vi "POSITION ARM ANGLE.vi"(0 "ARM devref in":T1={"DeviceStatus"={"status"=FALSE, "code"=0, "source"=""}, "Type"=enum."PWM", "PWM"={"PWM Channel"=enum."Invalid", "DeadBand"={"Name"="", "maxPositivePwm"=0, "minPositivePwm"=0, "centerPwm"=0, "maxNegativePwm"=0, "minNegativePwm"=0, "angularRange"=0}}, "CAN"={"Device Number"=0, "SetOutput VI Ref"=variant, "GetOutput VI Ref"=variant, "Enable VI Ref"=variant, "Disable VI Ref"=variant, "Data"=variant}, "Invert"=FALSE, "DIO PWM"={"PWM \"Enable\" Channel"=enum."Invalid", "DIOChannel"=enum."Invalid", "PWM Rate"=0.0}}, 1 "LEFT-RIGHT":string="LEFT", 2 "Setpoint":dbl=515.0, 5 "error in (no error)":errorcluster, 7 "PID Constants":T6={"P Gain"=2.0599999999999987, "I Gain"=0.0, "D Gain"=0.20000000000000004, "F Gain"=0.0, "I Zone"=0.0, "Min Output"=-0.1999999999999993, "Max Output"=0.95} {"Max Output" min=-1.0 max=1.0 step=0.01; "Min Output" min=-1.0 max=1.0 step=0.01; "I Zone" step=0.01; "F Gain" step=0.01; "D Gain" step=0.01; "I Gain" step=0.01; "P Gain" min=0.0 step=0.01}) -> (14 "Position":dbl, 16 "Output":dbl, 19 "error out":errorcluster)   [LabVIEW 2020]
uses:
  <vilib>/Rock Robotics/WPI/MotorControl/WPI_MotorControlDeviceRef.ctl
  <vilib>/Rock Robotics/WPI/MotorControl/WPI_MotorControlType.ctl
  <vilib>/Rock Robotics/SystemInterfaces/DIO/FPGA_DIOPWMChannel.ctl
  <vilib>/Rock Robotics/WPI/PWM/WPI_PWMDeadband.ctl
  <vilib>/Rock Robotics/SystemInterfaces/DIO/FPGA_DIOChannel.ctl
  <vilib>/Rock Robotics/WPI/ThirdParty/REV Robotics/REVLib/Typedef/Spark MAX Control Type.ctl
  Robot Global Data.vi
  <vilib>/Rock Robotics/Network Tables/NT Read Number.vi
panel:
  in  "NT arm string":string="ARM"
  in  "nt set pos string":string="/setPOS"
  out "MotorControlDevRef out":T1={"DeviceStatus"={"status"=FALSE, "code"=0, "source"=""}, "Type"=enum."PWM", "PWM"={"PWM Channel"=enum."Invalid", "DeadBand"={"Name"="", "maxPositivePwm"=0, "minPositivePwm"=0, "centerPwm"=0, "maxNegativePwm"=0, "minNegativePwm"=0, "angularRange"=0}}, "CAN"={"Device Number"=0, "SetOutput VI Ref"=variant, "GetOutput VI Ref"=variant, "Enable VI Ref"=variant, "Disable VI Ref"=variant, "Data"=variant}, "Invert"=FALSE, "DIO PWM"={"PWM \"Enable\" Channel"=enum."Invalid", "DIOChannel"=enum."Invalid", "PWM Rate"=0.0}}
  out "PID Chart":T7(graph)
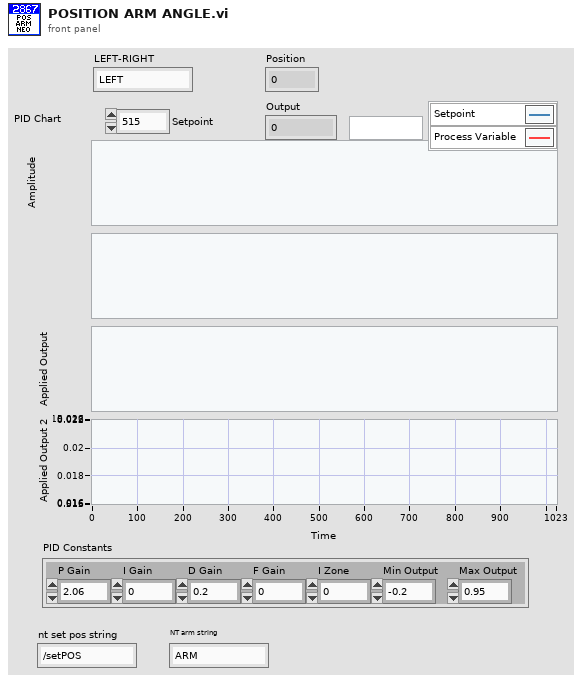
[diagram p1: front panel]
types:
  T1 = typedef "WPI_MotorControlDeviceRef.ctl" = cluster{"DeviceStatus":errorcluster, "Type":T2, "PWM":cluster{"PWM Channel":T3, "DeadBand":T4}, "CAN":cluster{"Device Number":u8, "SetOutput VI Ref":variant, "GetOutput VI Ref":variant, "Enable VI Ref":variant, "Disable VI Ref":variant, "Data":variant}, "Invert":bool, "DIO PWM":cluster{"PWM \"Enable\" Channel":T3, "DIOChannel":T5, "PWM Rate":dbl}}
  T2 = typedef "WPI_MotorControlType.ctl" = enum16{"PWM", "CAN", "DIO PWM"}
  T3 = typedef "FPGA_DIOPWMChannel.ctl" = enum8{"PWM 0", "PWM 1", "PWM 2", "PWM 3", "PWM 4", "PWM 5", "PWM 6", "PWM 7", "PWM 8", "PWM 9", "PWM MXP 0", "PWM MXP 1", "PWM MXP 2", "PWM MXP 3", "PWM MXP 4", "PWM MXP 5", "PWM MXP 6", "PWM MXP 7", "PWM MXP 8", "PWM MXP 9", "Invalid"}
  T4 = typedef "WPI_PWMDeadband.ctl" = cluster{"Name":string, "maxPositivePwm":i32, "minPositivePwm":i32, "centerPwm":i32, "maxNegativePwm":i32, "minNegativePwm":i32, "angularRange":u16}
  T5 = typedef "FPGA_DIOChannel.ctl" = enum8{"DIO 0", "DIO 1", "DIO 2", "DIO 3", "DIO 4", "DIO 5", "DIO 6", "DIO 7", "DIO 8", "DIO 9", "DIO MXP 0", "DIO MXP 1", "DIO MXP 2", "DIO MXP 3", "DIO MXP 4", "DIO MXP 5", "DIO MXP 6", "DIO MXP 7", "DIO MXP 8", "DIO MXP 9", "DIO MXP 10", "DIO MXP 11", "DIO MXP 12", "DIO MXP 13", "DIO MXP 14", "DIO MXP 15", "SPI Port CS1", "SPI Port CS2", "SPI Port CS3", "SPI Port MISO", "SPI Port MOSI", "Invalid"}
  T6 = cluster{"P Gain":dbl, "I Gain":dbl, "D Gain":dbl, "F Gain":dbl, "I Zone":dbl, "Min Output":dbl, "Max Output":dbl}
  T7 = cluster{"Sensor Position":dbl, "Sensor Position":dbl, "Setpoint":dbl, "Applied Output":dbl}
  T8 = cluster{"MIN":dbl, "MAX":dbl, "convert arm inches to revs":dbl}
  T9 = typedef "Spark MAX Control Type.ctl" = enum16{"Percent VBus", "Voltage", "Velocity", "Position", "Smart Motion", "Current", "Smart Velocity"}
  T10 = cluster{"P Gain":bool, "I Gain":bool, "D Gain":bool, "F Gain":bool, "I Zone":bool, "Min Output":bool, "Max Output":bool}
  T11 = typedef "Spark MAX Status 0 Frame.ctl" = cluster{"Applied Output":dbl, "Faults":T12, "Sticky Faults":T12, "Rsvd":u8, "Status 0 Flags":T13, "Timestamp":u32}
  T12 = typedef "Spark MAX Faults.ctl" = cluster{"Hard Limit Rev":bool, "Hard Limit Fwd":bool, "Soft Limit Fwd":bool, "Soft Limit Rev":bool, "Other Fault":bool, "DRV Fault":bool, "Has Reset?":bool, "CAN RX":bool, "CAN TX":bool, "EEPROM CRC":bool, "Stall":bool, "Sensor Fault":bool, "Motor Type Fault":bool, "IWDT Reset":bool, "Over Current":bool, "Brownout":bool}
  T13 = typedef "Spark MAX Status 0 Flags.ctl" = cluster{"Invert/Brake":bool, "Is Follower":bool}
  T14 = typedef "Spark MAX Status 2 Frame.ctl" = cluster{"Sensor Position":dbl, "IAccum":dbl, "Timestamp":u32}
  T15 = cluster{"Sensor Position":dbl, "Sensor Position":dbl, dbl, "Applied Output":dbl}
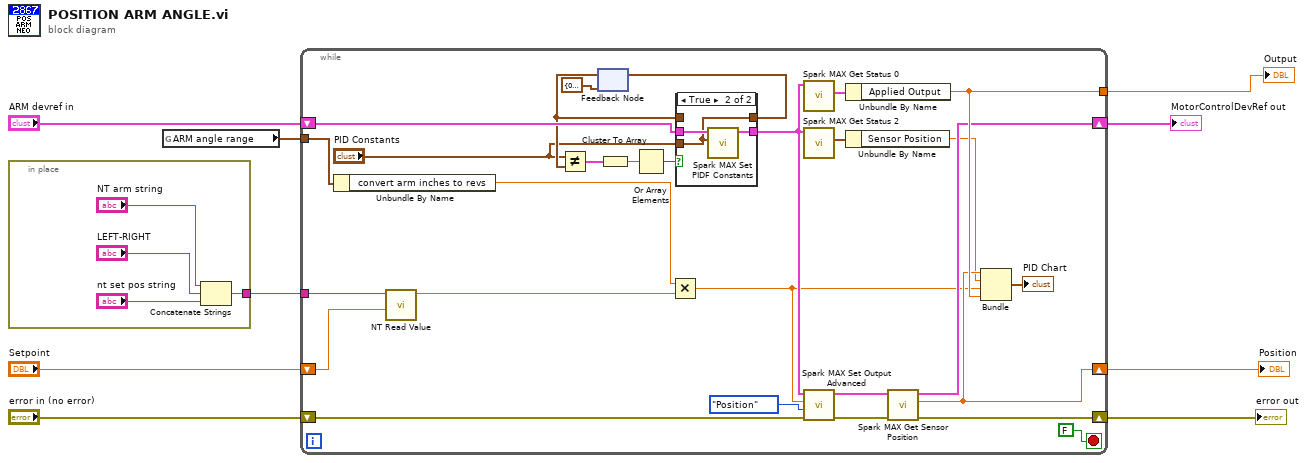
[diagram p0: block diagram]
diagram:
  n1 = in-place {
    in-place-border: [w10] -> w1
    n2 = Concatenate Strings("NT arm string", "LEFT-RIGHT", "nt set pos string") -> (w10:string)
  }
  n3 = global read "Robot Global Data.vi" "ARM angle range"() -> (w2:T8)
  n4 = while {
    tunnel: [w40] -> w7
    shift-right: [w41] -> w8
    shift-left: "error in (no error)" -> [w39]
    shift-right: [w36] -> w3
    shift-left: "ARM devref in" -> [w38]
    shift-right: [w37] -> w4
    shift-left: "Setpoint" -> [w14]
    tunnel: w2 -> [w26]
    tunnel: w1 -> [w25]
    stop <- FALSE stop-if-true
    n5 = Unbundle By Name(w26) -> ("convert arm inches to revs"=w23:dbl)
    n6 = call-poly <vilib>:"NT Read Value.vi"("Default Value"=w14, "Name"=w25) -> ("Numeric"=w24:dbl)  [unwired: 8 in, 1 out]
    n7 = feedback #1(T6 {"P Gain"=0.0, "I Gain"=0.0, "D Gain"=0.0, "F Gain"=0.0, "I Zone"=0.0, "Min Output"=0.0, "Max Output"=0.0} ("PID Constants")) -> (w21:T6)
    n8 = Not Equal?(x="PID Constants", y=w21) -> (x != y?=w16:T10)
    n9 = Cluster To Array(cluster=w16) -> (array=w17:bool[])
    n10 = Or Array Elements(Boolean array=w17) -> (logical OR=w19:bool)
    n11 = Multiply(x=w23, y=w24) -> (x*y=w22:dbl)
    n12 = case shown="True" w19 {
      tunnel: w38 -> [w42 w46]
      tunnel: "PID Constants" -> [_ w44]
      tunnel: [w43 w44] -> w20
      tunnel: w21 -> [w43 _]
      tunnel: [w42 w45] -> w31
      frame False {
      }
      frame True {
        n13 = call <vilib>:"Spark MAX Set PIDF Constants.vi"("PID Constants"=w44, "MotorControlDeviceRef"=w46) -> ("MotorControlDeviceRef"=w45:T1)  [unwired: 8 in, 1 out]
      }
    }
    n14 = feedback-in #1(w20) -> ()
    n15 = call <vilib>:"Spark MAX Get Status 0.vi"("MotorControlDevRef"=w31) -> ("Status 0"=w35:T11)  [unwired: 7 in, 3 out]
    n16 = call <vilib>:"Spark MAX Get Status 2.vi"("MotorControlDevRef"=w31) -> ("Stat 2"=w30:T14)  [unwired: 7 in, 3 out]
    n17 = call <vilib>:"Spark MAX Set Output Advanced.vi"("error in (no error)"=w39, "Control Mode"=Spark_MAX_Control_Type."Position", "Setpoint"=w22, "MotorControlDevRef"=w31) -> ("error out"=w28:errorcluster, "MotorControlDevRef"=w29:T1)  [unwired: 6 in]
    n18 = Unbundle By Name(w35) -> ("Applied Output"=w40:dbl)
    n19 = Unbundle By Name(w30) -> ("Sensor Position"=w32:dbl)
    n20 = call <vilib>:"Spark MAX Get Sensor Position.vi"("error in (no error)"=w28, "MotorControlDevRef in"=w29) -> ("error out"=w41:errorcluster, "Sensor Position"=w37:dbl, "MotorControlDevRef out"=w36:T1)  [unwired: 6 in, 1 out]
    n21 = Bundle("Sensor Position"=w37, "Sensor Position"=w32, w22, "Applied Output"=w40) -> (→"PID Chart":T15)  [unwired: 1 in]
  }
  "Output" <- w7
  "error out" <- w8
  "Position" <- w4
  "MotorControlDevRef out" <- w3
